vi "check if odd or even.vi"(11 "int":i32) -> (3 "even?":bool)   [LabVIEW 2018]
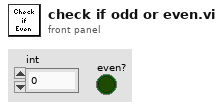
[diagram p1: front panel]
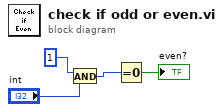
[diagram p0: block diagram]
diagram:
  n1 = And(x=1, y="int") -> (x .and. y?=w3:i32)
  n2 = Equal To 0?(x=w3) -> (x = 0?=→"even?":bool)
